vi "Precision_RFS.vi"(6 "Type y_pred":T1(ring), 7 "Type y_true":T1(ring), 8 "error in (no error)":errorcluster caption="entrée d'erreur (pas d'erreur)", 9 "y_pred":string[][](array[string]), 10 "y_true":string[][](array[string]), 11 "precision_recall_fscore_support":T3={"beta"=1.0, "labels"=["None"], "pos_label"={"dtype_pos_label"="int", "pos_label"="1"}, "average"="None", "warn_for"=["precision", "recall", "f-score"], "sample_weight"=[], "zero_division"={"dtype_zero_division"="str", "zero_division"="warn"}, "Returns"="precision"}) -> (0 "error out":errorcluster caption="sortie d'erreur", 3 "Data":T2)   [LabVIEW 2020]
doc: "Compute precision, recall, F-measure and support for each class\n\nThe precision is the ratio tp / (tp + fp) where tp is the number of true positives and fp the number of false positives. The precision is intuitively the ability of the classifier not to label as positive a sample that is negative.\n\nThe recall is the ratio tp / (tp + fn) where tp is the number of true positives and fn the number of false negatives. The recall is intuitively the ability of the classifier to find all the positive samples.\n\nThe F-beta score can be interpreted as a weighted harmonic mean of the precision and recall, where an F-beta score reaches its best value at 1 and worst score at 0.\n\nThe F-beta score weights recall more than precision by a factor of beta. beta == 1.0 means recall and precision are equally important.\n\nThe support is the number of occurrences of each class in y_true.\n\nIf pos_label is None and in binary classification, this function returns the average precision, recall and F-measure if average is one of 'micro', 'macro', 'weighted' or 'samples'.\n\n\n\nParameters : \n\n- y_true : 1d array-like, or label indicator array / sparse matrix\nGround truth (correct) target values.\n\n- y_pred : 1d array-like, or label indicator array / sparse matrix\nEstimated targets as returned by a classifier.\n\n- beta : float, 1.0 by default\nThe strength of recall versus precision in the F-score.\n\n- labels : list, optional\nThe set of labels to include when average != 'binary', and their order if average is None. Labels present in the data can be excluded, for example to calculate a multiclass average ignoring a majority negative class, while labels not present in the data will result in 0 components in a macro average. For multilabel targets, labels are column indices. By default, all labels in y_true and y_pred are used in sorted order.\n\n- pos_label : str or int, 1 by default\nThe class to report if average='binary' and the data is binary. If the data are multiclass or multilabel, this will be ignored; setting labels=[pos_label] and average != 'binary' will report scores for that label only.\n\n- average : string, [None (default), ‘binary’, ‘micro’, ‘macro’, ‘samples’, ‘weighted’]\nIf None, the scores for each class are returned. Otherwise, this determines the type of averaging performed on the data:\n\n'binary':\nOnly report results for the class specified by pos_label. This is applicable only if targets (y_{true,pred}) are binary.\n\n'micro':\nCalculate metrics globally by counting the total true positives, false negatives and false positives.\n\n'macro':\nCalculate metrics for each label, and find their unweighted mean. This does not take label imbalance into account.\n\n'weighted':\nCalculate metrics for each label, and find their average weighted by support (the number of true instances for each label). This alters ‘macro’ to account for label imbalance; it can result in an F-score that is not between precision and recall.\n\n'samples':\nCalculate metrics for each instance, and find their average (only meaningful for multilabel classification where this differs from accuracy_score).\n\n- warn_for : tuple or set, for internal use\nThis determines which warnings will be made in the case that this function is being used to return only one of its metrics.\n\n- sample_weight : array-like of shape (n_samples,), default=None\nSample weights.\n\n- zero_division : “warn”, 0 or 1, default=”warn”\nSets the value to return when there is a zero division :\n recall : when there are no positive labels\n precision : when there are no positive predictions\n f-score : both\n\nIf set to “warn”, this acts as 0, but warnings are also raised.\n\nReturns : \n\n- precision : float (if average is not None) or array of float, shape = [n_unique_labels]\n- recall : float (if average is not None) or array of float, , shape = [n_unique_labels]\n- fbeta_score : float (if average is not None) or array of float, shape = [n_unique_labels]\n- support : None (if average is not None) or array of int, shape = [n_unique_labels]\n The number of occurrences of each label in y_true."
uses:
  Precision_RFS.lvclass
panel:
  out "Precision_RFS.lvclass":refnum<class "Precision_RFS.lvclass">
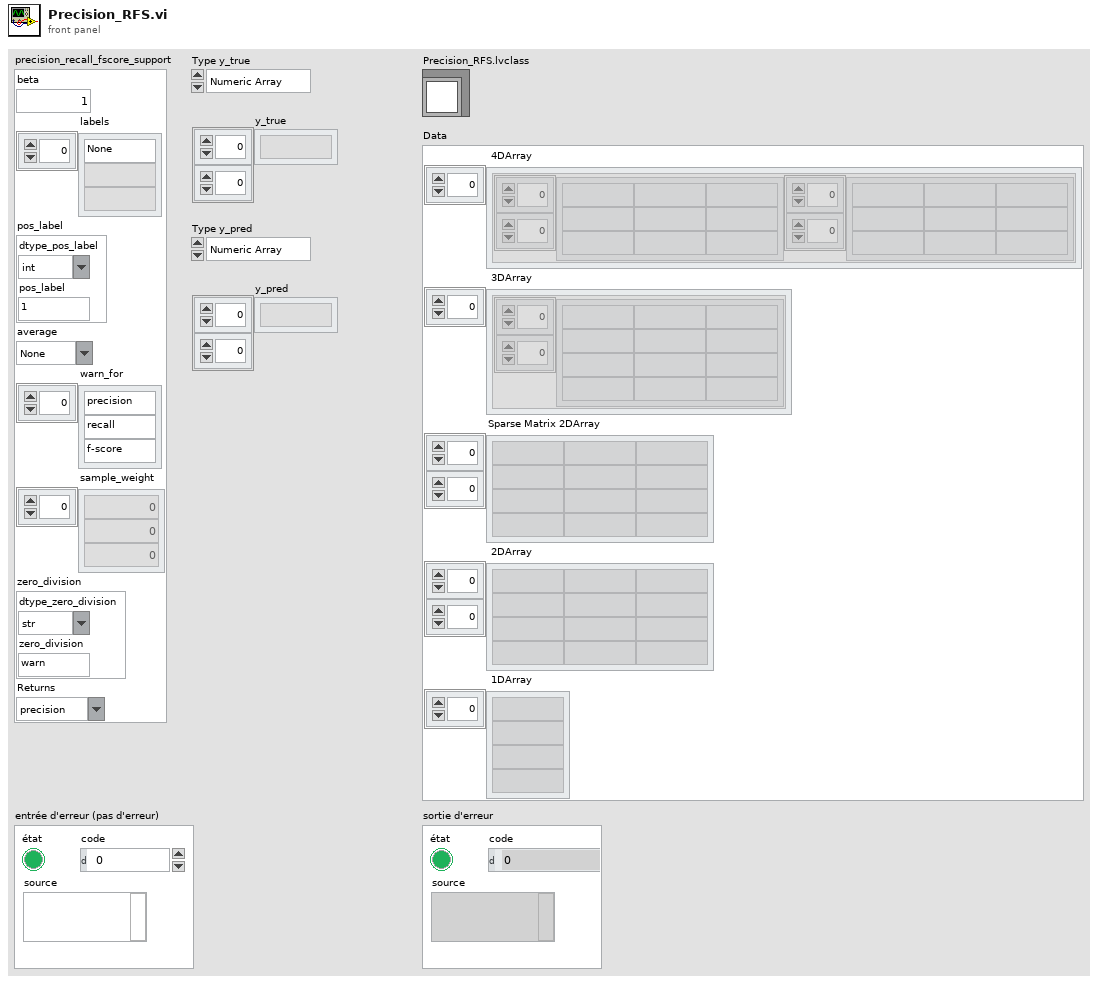
[diagram p1: front panel]
types:
  T1 = enum16{"Numeric Array", "String Array", "Sparse"}
  T2 = cluster{" 4DArray":cluster{"1":string[][], "2":string[][]}[], " 3DArray":cluster{"Tableau":string[][]}[], "Sparse Matrix 2DArray":string[][], " 2DArray":string[][], " 1DArray":string[]}
  T3 = cluster{"beta":dbl, "labels":string[], "pos_label":cluster{"dtype_pos_label":string, "pos_label":string}, "average":string, "warn_for":string[], "sample_weight":dbl[], "zero_division":cluster{"dtype_zero_division":string, "zero_division":string}, "Returns":string}
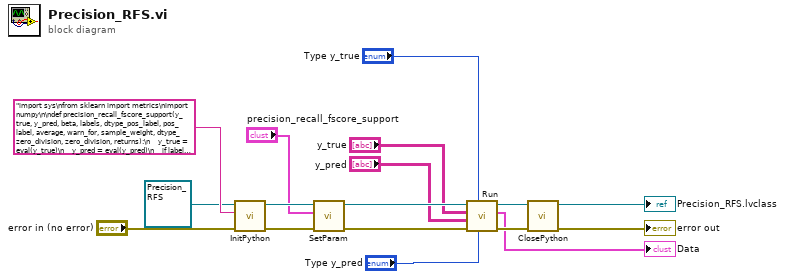
[diagram p0: block diagram]
diagram:
  n1 = call-dynamic "InitPython.vi"("error in (no error)"="error in (no error)", "Python Instruction"="import sys\nfrom sklearn import metrics\nimport numpy\n\ndef precision_recall_fscore_support(y_true, y_pred, beta, labels, dtype_pos_label, pos_label, average, warn_for, sample_weight, dtype_zero_division, zero_division, returns):\n    y_true = eval(y_true)\n    y_pred = eval(y_pred)\n    if labels == [] or labels[0] == 'None':\n        labels = None\n    if dtype_pos_label == 'int':\n        pos_label = eval(pos_label)\n    if average == 'None':\n        average = None\n    if sample_weight == []:\n        sample_weight = None\n    if dtype_zero_division == 'int':\n        zero_division = eval(zero_division)\n    try:\n        precision, recall, fbeta_score, support = metrics.precision_recall_fscore_support(y_true, y_pred, beta, labels, pos_label, average, warn_for, sample_weight, zero_division)\n        if returns == 'precision':\n            precision_recall_fscore_support = precision.tolist()\n            return str(precision_recall_fscore_support)\n        elif returns == 'recall':\n            precision_recall_fscore_support = recall.tolist()\n            return str(precision_recall_fscore_support)\n        elif returns == 'fbeta_score':\n            precision_recall_fscore_support = fbeta_score.tolist()\n            return str(precision_recall_fscore_support)\n        else: \n            precision_recall_fscore_support = support.tolist()\n            return str(precision_recall_fscore_support)\n    except:\n        erreur = sys.exc_info()\n        typerr = u\"%s\" % (erreur[0])\n        typerr = typerr[typerr.find(\"'\")+1:typerr.rfind(\"'\")]\n        msgerr = u\"%s\" % (erreur[1])\n        message = str('/!\\\\ {0} : {1}'. format(typerr,msgerr))\n        return message", "Scikit-learn en entrée"=refnum<class "Precision_RFS.lvclass"> refnum ("Precision_RFS.lvclass")) -> ("error out"=w13:errorcluster, "Scikit-learn en sortie"=w15:refnum<class "Precision_RFS.lvclass">)  [unwired: 7 in]
  n2 = call-dynamic "SetParam.vi"("error in (no error)"=w13, "precision_recall_fscore_support"="precision_recall_fscore_support", "Precision_RFS.lvclass"=w15) -> ("error out"=w11:errorcluster, "Precision_RFS.lvclass"=w12:refnum<class "Precision_RFS.lvclass">)  [unwired: 7 in]
  n3 = call-dynamic "Run.vi"("Type y_pred"="Type y_pred", "Type y_true"="Type y_true", "error in (no error)"=w11, "y_pred"="y_pred", "y_true"="y_true", "Precision_RFS.lvclass"=w12) -> ("error out"=w10:errorcluster, "Data"=→"Data":T2, "Precision_RFS.lvclass"=w9:refnum<class "Precision_RFS.lvclass">)  [unwired: 3 in]
  n4 = call-dynamic "ClosePython.vi"("error in (no error)"=w10, "Scikit-learn en entrée"=w9) -> ("error out"=→"error out":errorcluster, "Scikit-learn en sortie"=→"Precision_RFS.lvclass":refnum<class "Precision_RFS.lvclass">)  [unwired: 8 in]
